vi "Check Template Consistency.vi"(11 "Template Method Path":path) -> (2 "Template is OK?":bool)   [LabVIEW 2013, in "Scripter.lvlib"]
uses:
  Scripter.lvlib
  <vilib>/Utility/traverseref.llb/TRef TravTarget.ctl
  <vilib>/Utility/traverseref.llb/VI Scripting - Traverse.lvlib
panel:
  out "Error Out":errorcluster
  in  "Error In":errorcluster
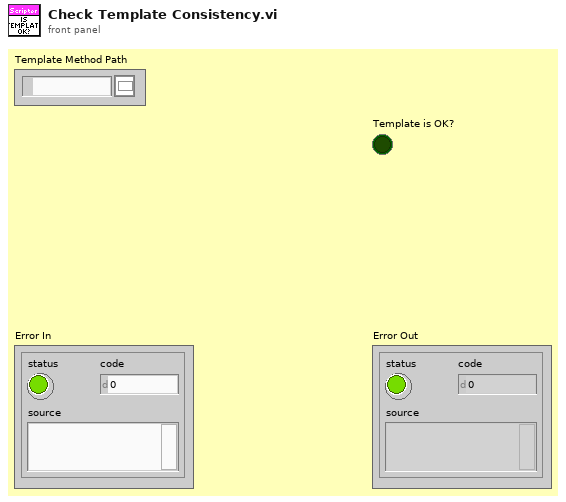
[diagram p1: front panel]
types:
  T1 = typedef "TRef TravTarget.ctl" = enum16{"FP", "BD", "Other"}
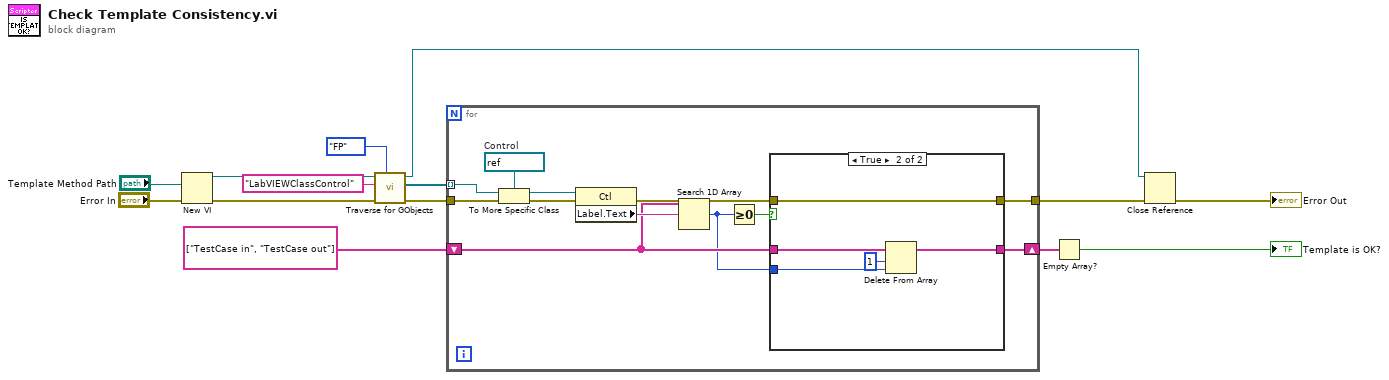
[diagram p0: block diagram]
diagram:
  n1 = New VI(8:"Error In", 10:"Template Method Path") -> (0:w13:errorcluster, 3:w8:refnum<vi>)  [unwired: 5 in]
  n2 = call <vilib>:"Traverse for GObjects.vi"("Traverse Target"=TRef_TravTarget."FP", "error in (no error)"=w13, "Class Name"="LabVIEWClassControl", "VI Refnum"=w8) -> ("error out"=w9:errorcluster, "References"=w5:refnum<vi>[], "dup VI Refnum"=w6:refnum<vi>)  [unwired: 4 in, 1 out]
  n3 = for {
    tunnel: w5 -> [w26] mode=indexing
    tunnel: w9 -> [w22]
    tunnel: [w18] -> w7
    shift-right: [w16] -> w3
    shift-left: string[] ["TestCase in", "TestCase out"] -> [w17]
    w24 = refnum<vi> refnum  # Control
    n4 = To More Specific Class(target class=w24, reference=w26, error in=w22) -> (specific class reference=w25:refnum<vi>, error out=w21:errorcluster)
    n5 = property class="Ctl"(reference=w25, error in=w21) -> (error out=w19:errorcluster, "Label.Text"=w23:string)  [unwired: 1 out]
    n6 = Search 1D Array(1D array=w17, element=w23) -> (index of element=w15:i32)  [unwired: 1 in]
    n7 = Greater Or Equal To 0?(x=w15) -> (x >= 0?=w20:bool)
    n8 = case shown="True" w20 {
      tunnel: w19 -> [w28 w33]
      tunnel: [w28 w33] -> w18
      tunnel: w17 -> [w27 w32]
      tunnel: [w27 w31] -> w16
      tunnel: w15 -> [_ w30]
      frame False {
      }
      frame True {
        n9 = Delete From Array(array=w32, length=1, index=w30) -> (array with subset deleted=w31:string[])  [unwired: 1 out]
      }
    }
  }
  n10 = Empty Array?(array=w3) -> (empty?=→"Template is OK?":bool)
  n11 = Close Reference(reference=w6, error in (no error)=w7) -> (error out=→"Error Out":errorcluster)
